vi "Plot Editor_Store to Controls.vi"(8 "Error In":errorcluster, 10 "Control Refnums":refnum<vi>[](array[refnum]), 11 "Plot Editor Internal Data in":T1) -> (0 "Error Out":errorcluster, 3 "Plot Editor Internal Data out":T1)   [LabVIEW 2019, in "Plot Editor.lvlib"]
uses:
  Plot Editor.lvlib
  Plot Editor Internal Variables.ctl
  XY Graph/XY Graph Plot Properties.ctl
panel:
  in  "DBL Numeric":refnum<vi>
  in  "Array":refnum<vi>
  in  "I32 Numeric":refnum<vi>
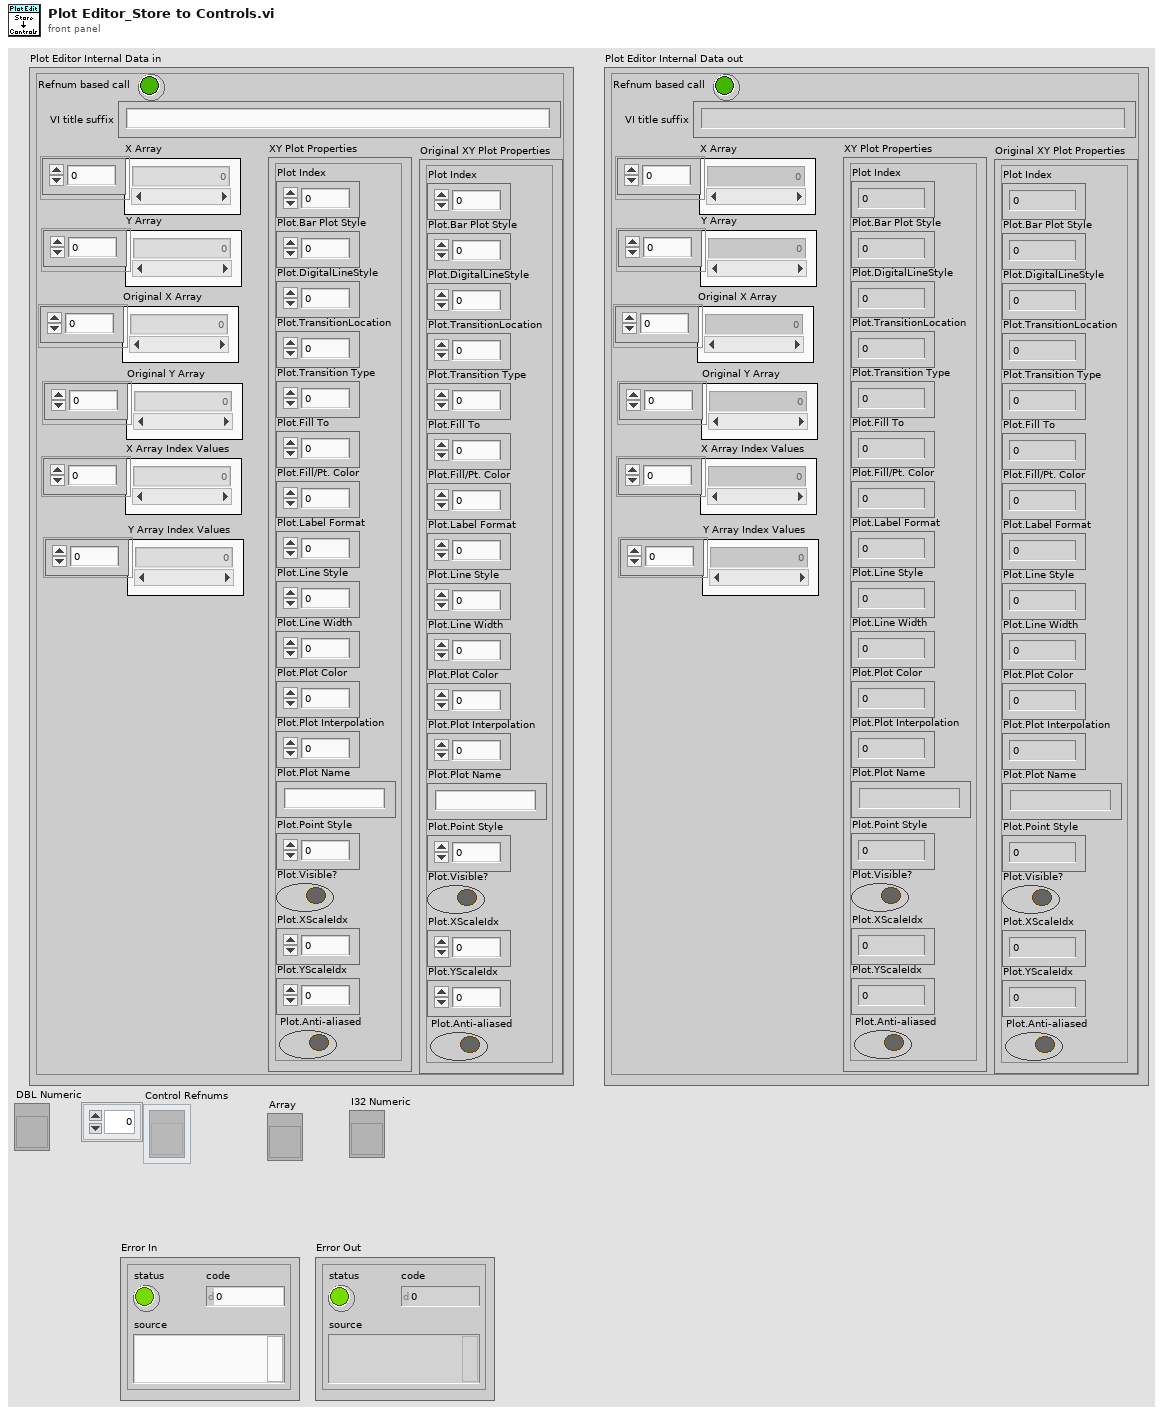
[diagram p1: front panel]
types:
  T1 = typedef "Plot Editor.lvlib/Plot Editor Internal Variables.ctl" = cluster{"X Array":dbl[], "Y Array":dbl[], "XY Plot Properties":T2, "X Array Index Values":u32[], "Y Array Index Values":u32[], "Original XY Plot Properties":T2, "Original X Array":dbl[], "Original Y Array":dbl[], "VI title suffix":string, "Refnum based call":bool}
  T2 = typedef "XY Graph Plot Properties.ctl" = cluster{"Plot Index":i32, "Plot.Bar Plot Style":u8, "Plot.DigitalLineStyle":u8, "Plot.TransitionLocation":u8, "Plot.Transition Type":u8, "Plot.Fill To":i16, "Plot.Fill/Pt. Color":u32, "Plot.Label Format":u8, "Plot.Line Style":u8, "Plot.Line Width":u8, "Plot.Plot Color":u32, "Plot.Plot Interpolation":u8, "Plot.Plot Name":string, "Plot.Point Style":u8, "Plot.Visible?":bool, "Plot.XScaleIdx":u32, "Plot.YScaleIdx":u32, "Plot.Anti-aliased":bool}
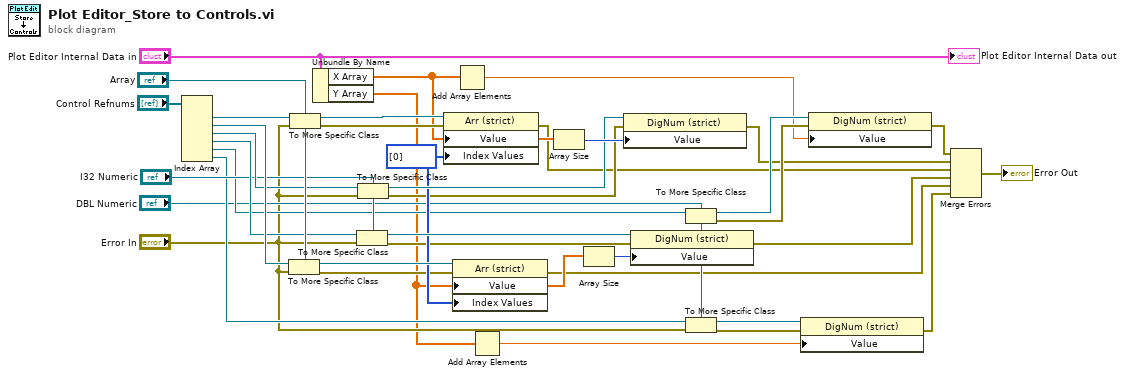
[diagram p0: block diagram]
diagram:
  w23 = u32[] [0] ("Index Values")
  n1 = Index Array(array="Control Refnums") -> (element #1=w35:refnum<vi>, element #2=w33:refnum<vi>, element #3=w30:refnum<vi>, element #4=w28:refnum<vi>, element #5=w21:refnum<vi>, element #6=w10:refnum<vi>)  [unwired: 6 in]
  n2 = To More Specific Class(target class="Array", reference=w33, error in="Error In") -> (specific class reference=w31:refnum<vi>, error out=w17:errorcluster)
  n3 = To More Specific Class(target class="Array", reference=w35, error in="Error In") -> (specific class reference=w34:refnum<vi>, error out=w18:errorcluster)
  n4 = Unbundle By Name("Plot Editor Internal Data in") -> ("X Array"=w14:dbl[], "Y Array"=w5:dbl[])
  n5 = To More Specific Class(target class="I32 Numeric", reference=w28, error in="Error In") -> (specific class reference=w26:refnum<vi>, error out=w16:errorcluster)
  n6 = To More Specific Class(target class="I32 Numeric", reference=w30, error in="Error In") -> (specific class reference=w29:refnum<vi>, error out=w19:errorcluster)
  n7 = property class="Arr (strict)"(reference=w34, error in=w18, "Value"=w14, "Index Values"=w23) -> (error out=w11:errorcluster)  [unwired: 1 out]
  n8 = property class="Arr (strict)"(reference=w31, error in=w17, "Value"=w5, "Index Values"=w23) -> (error out=w2:errorcluster)  [unwired: 1 out]
  n9 = Add Array Elements(numeric array=w14) -> (sum=w13:dbl)
  n10 = Add Array Elements(numeric array=w5) -> (sum=w4:dbl)
  n11 = Array Size(array=w14) -> (size(s)=w37:i32)
  n12 = Array Size(array=w5) -> (size(s)=w38:i32)
  n13 = property class="DigNum (strict)"(reference=w29, error in=w19, "Value"=w37) -> (error out=w12:errorcluster)  [unwired: 1 out]
  n14 = property class="DigNum (strict)"(reference=w26, error in=w16, "Value"=w38) -> (error out=w3:errorcluster)  [unwired: 1 out]
  n15 = To More Specific Class(target class="DBL Numeric", reference=w21) -> (specific class reference=w20:refnum<vi>, error out=w15:errorcluster)  [unwired: 1 in]
  n16 = To More Specific Class(target class="DBL Numeric", reference=w10, error in="Error In") -> (specific class reference=w7:refnum<vi>, error out=w6:errorcluster)
  n17 = property class="DigNum (strict)"(reference=w7, error in=w6, "Value"=w4) -> (error out=w1:errorcluster)  [unwired: 1 out]
  n18 = property class="DigNum (strict)"(reference=w20, error in=w15, "Value"=w13) -> (error out=w22:errorcluster)  [unwired: 1 out]
  n19 = Merge Errors(w22, w12, w11, w3, w2, w1) -> (→"Error Out":errorcluster)
  "Plot Editor Internal Data out" <- "Plot Editor Internal Data in"
